vi "PCO_RebootCamera.vi"(8 "error in (no error)":errorcluster {"code" format="%x"}, 11 "ph":u64) -> (0 "error out":errorcluster {"code" format="%x"}, 2 "ErrorMessage":i32 format="%x", 3 "ph out":u64)   [LabVIEW 2019, in "SDK.lvlib" / "GeneralCameraControl.lvlib"]
doc: "<b>Description:</b>\nThis function will reboot the camera. The function will return immediately and the reboot process in the camera is started. After calling this command the handle to this camera should be closed with PCO_CloseCamera.\nWhen reboot is finished (approximately after 6 to 10 seconds, up to 40 seconds for cameras with GigE interface) the camera can be reopened with a PCO_OpenCameraEx call. The reboot command is used during firmware update and is necessary when camera setup is changed.\n\n<b>Supported camera type:</b>\nAll cameras\n\n<b>Descriptor dependency:</b>\nNone"
uses:
  GeneralCameraControl.lvlib
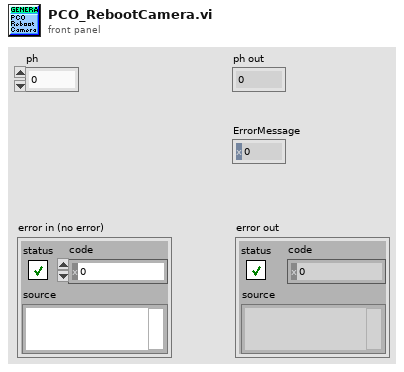
[diagram p1: front panel]
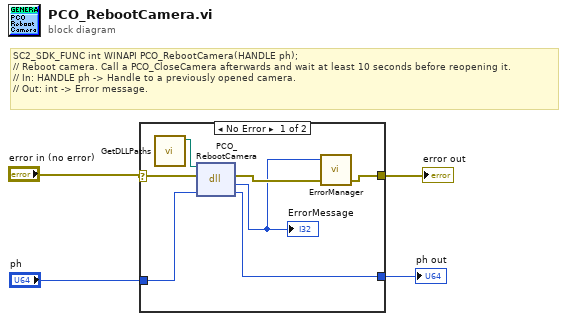
[diagram p0: block diagram]
diagram:
  # "SC2_SDK_FUNC int WINAPI PCO_RebootCamera(HANDLE ph);\n// Reboot camera. Call a PCO_CloseCamera afterwards and wait at least 10 seconds before reopening it.\n// In: HANDLE ph -> Handle to a previously opened camera.\n// Out: int -> Error message."
  n1 = case shown="No Error" "error in (no error)" {
    selector: "error in (no error)" -> [w9 w12]
    tunnel: "ph" -> [w11 w13]
    tunnel: [w10 w13] -> w3
    tunnel: [w7 w12] -> w1
    frame No Error {
      n2 = call "GetDLLPaths.vi"() -> ("SC2_Cam_Path"=w5:path)  [unwired: 9 in, 2 out]
      n3 = dll-call lib="?" fn="PCO_RebootCamera"(path in=w5, error in=w9, "ph"=w11) -> (error out=w8:errorcluster, "return type"=w6:i32, "ph"=w10:u64)  [unwired: 1 in, 1 out]
      "ErrorMessage" <- w6
      n4 = call "ErrorManager.vi"("error in (no error)"=w8, "error code"=w6) -> ("error out"=w7:errorcluster)  [unwired: 3 in]
    }
    frame Error {
    }
  }
  "ph out" <- w3
  "error out" <- w1
